vi "CameraCheckROI.vi"(8 "error in (no error)":errorcluster, 10 "ROI_in":T1, 11 "CameraBase in":refnum<class "CameraBase.lvclass">) -> (0 "error out":errorcluster, 2 "ROI_out":T1, 3 "CameraBase out":refnum<class "CameraBase.lvclass">)   [LabVIEW 2010, in "CameraBase.lvclass"]
uses:
  CameraBase.lvclass
  subvis/ROI_rect.ctl
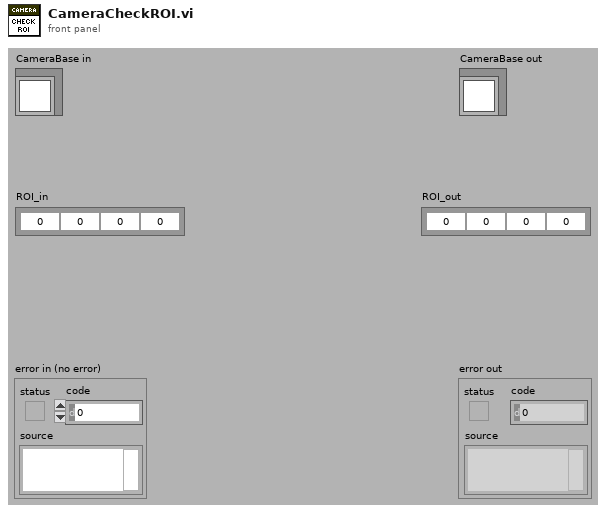
[diagram p1: front panel]
types:
  T1 = typedef "ROI_rect.ctl" = cluster{"left":i32, "top":i32, "right":i32, "bottom":i32}
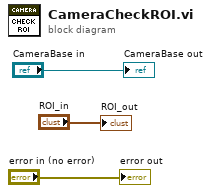
[diagram p0: block diagram]
diagram:
  "error out" <- "error in (no error)"
  "CameraBase out" <- "CameraBase in"
  "ROI_out" <- "ROI_in"
